vi "While Loop.vi"() -> ()   [LabVIEW 2015]
panel:
  in  "Condition Met?":bool
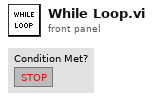
[diagram p1: front panel]
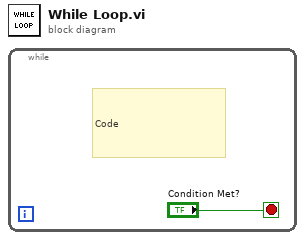
[diagram p0: block diagram]
diagram:
  n1 = while {
    stop <- "Condition Met?" stop-if-true
    # "Code"
  }
